vi "PicoScope4000aProbeInteraction.vi"(7 "Device Info":T2={"Driver Version"="2.1.44.2194", "USB Version"="3.0", "Hardware"="1", "Variant"="4444", "Batch and Serial"="FU827/0013", "Cal Date"="17Apr18", "Kernel Version"="1.0", "Digital HW Version"="1", "Analogue HW Version"="1", "Firmware 1"="1.7.5.0", "Firmware 2"="1.1.6.0", "Num. channels"=4}, 8 "error in":errorcluster, 11 "handle in":i16=16384) -> (0 "error out":errorcluster, 3 "handle out":i16=16384, 4 "Output Probe Array":T1(array[cluster])=[{"probeNumber"=0, FALSE, "channel"=-1, "enabled"=0, "probeName"=0, "requiresPower"=0, "isPowered"=0, "probeOff"=0, "rangeFirst"=0, "rangeLast"=0, "rangeCurrent"=0, "couplingFirst"=0, "couplingLast"=0, "couplingCurrent"=0, "filterFlags"=0, "filterCurrent"=0, "defaultFilter"=0}, {"probeNumber"=0, FALSE, "channel"=-1, "enabled"=0, "probeName"=0, "requiresPower"=0, "isPowered"=0, "probeOff"=0, "rangeFirst"=0, "rangeLast"=0, "rangeCurrent"=0, "couplingFirst"=0, "couplingLast"=0, "couplingCurrent"=0, "filterFlags"=0, "filterCurrent"=0, "defaultFilter"=0}, {"probeNumber"=0, FALSE, "channel"=-1, "enabled"=0, "probeName"=0, "requiresPower"=0, "isPowered"=0, "probeOff"=0, "rangeFirst"=0, "rangeLast"=0, "rangeCurrent"=0, "couplingFirst"=0, "couplingLast"=0, "couplingCurrent"=0, "filterFlags"=0, "filterCurrent"=0, "defaultFilter"=0}, {"probeNumber"=0, FALSE, "channel"=-1, "enabled"=0, "probeName"=0, "requiresPower"=0, "isPowered"=0, "probeOff"=0, "rangeFirst"=0, "rangeLast"=0, "rangeCurrent"=0, "couplingFirst"=0, "couplingLast"=0, "couplingCurrent"=0, "filterFlags"=0, "filterCurrent"=0, "defaultFilter"=0}], 6 "ProbeStateChanged":bool)   [LabVIEW 2010]
uses:
  ps4000aWrap.dll
panel:
  out "Probe Array Updates":T1(array[cluster])
  in  "Probe Input Array":T1(array[cluster])=[{"probeNumber"=0, FALSE, "channel"=-1, "enabled"=0, "probeName"=0, "requiresPower"=0, "isPowered"=0, "probeOff"=0, "rangeFirst"=0, "rangeLast"=0, "rangeCurrent"=0, "couplingFirst"=0, "couplingLast"=0, "couplingCurrent"=0, "filterFlags"=0, "filterCurrent"=0, "defaultFilter"=0}, {"probeNumber"=0, FALSE, "channel"=-1, "enabled"=0, "probeName"=0, "requiresPower"=0, "isPowered"=0, "probeOff"=0, "rangeFirst"=0, "rangeLast"=0, "rangeCurrent"=0, "couplingFirst"=0, "couplingLast"=0, "couplingCurrent"=0, "filterFlags"=0, "filterCurrent"=0, "defaultFilter"=0}, {"probeNumber"=0, FALSE, "channel"=-1, "enabled"=0, "probeName"=0, "requiresPower"=0, "isPowered"=0, "probeOff"=0, "rangeFirst"=0, "rangeLast"=0, "rangeCurrent"=0, "couplingFirst"=0, "couplingLast"=0, "couplingCurrent"=0, "filterFlags"=0, "filterCurrent"=0, "defaultFilter"=0}, {"probeNumber"=0, FALSE, "channel"=-1, "enabled"=0, "probeName"=0, "requiresPower"=0, "isPowered"=0, "probeOff"=0, "rangeFirst"=0, "rangeLast"=0, "rangeCurrent"=0, "couplingFirst"=0, "couplingLast"=0, "couplingCurrent"=0, "filterFlags"=0, "filterCurrent"=0, "defaultFilter"=0}]
  out "numberOfProbes":i32=1
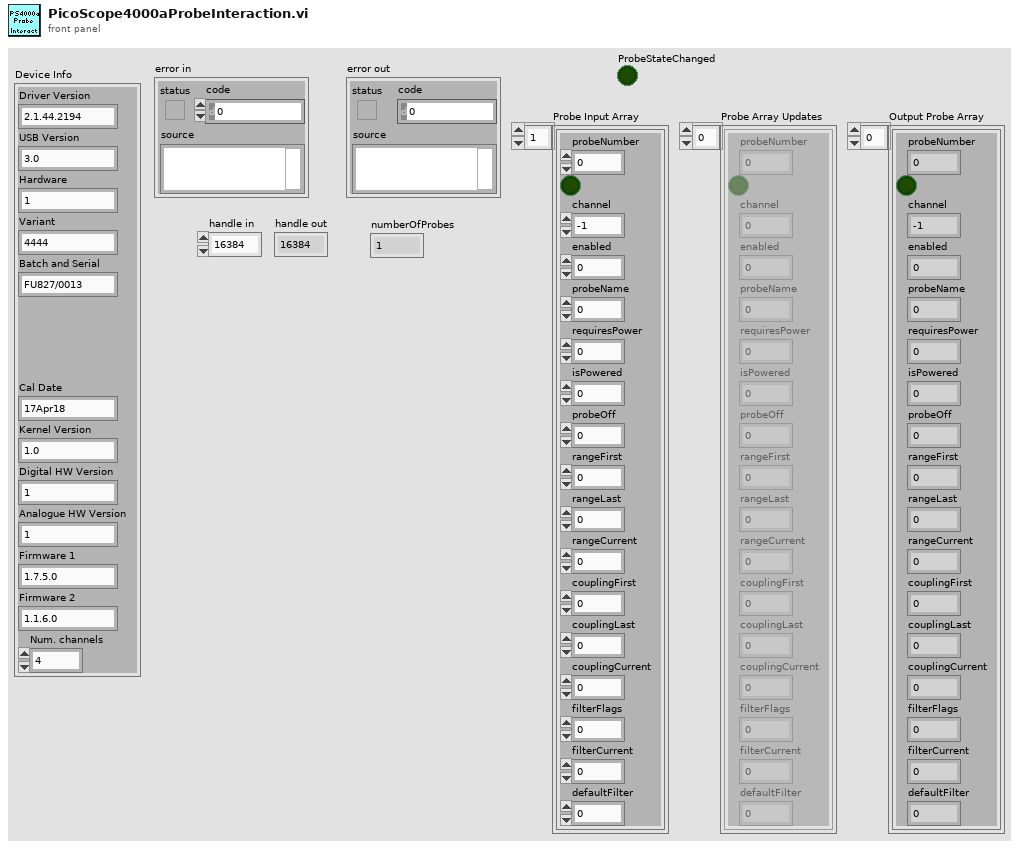
[diagram p1: front panel]
types:
  T1 = cluster{"probeNumber":i32, bool, "channel":i32, "enabled":i16, "probeName":i32, "requiresPower":i8, "isPowered":i8, "probeOff":i32, "rangeFirst":i32, "rangeLast":i32, "rangeCurrent":i32, "couplingFirst":i32, "couplingLast":i32, "couplingCurrent":i32, "filterFlags":i32, "filterCurrent":i32, "defaultFilter":i32}[]
  T2 = cluster{"Driver Version":string, "USB Version":string, "Hardware":string, "Variant":string, "Batch and Serial":string, "Cal Date":string, "Kernel Version":string, "Digital HW Version":string, "Analogue HW Version":string, "Firmware 1":string, "Firmware 2":string, "Num. channels":i16}
  T3 = cluster{"status":bool, "code":u32, "source":string}
  T4 = cluster{"probeNumber":i32, bool, "channel":i32, "enabled":i16, "probeName":i32, "requiresPower":i8, "isPowered":i8, "probeOff":i32, "rangeFirst":i32, "rangeLast":i32, "rangeCurrent":i32, "couplingFirst":i32, "couplingLast":i32, "couplingCurrent":i32, "filterFlags":i32, "filterCurrent":i32, "defaultFilter":i32}
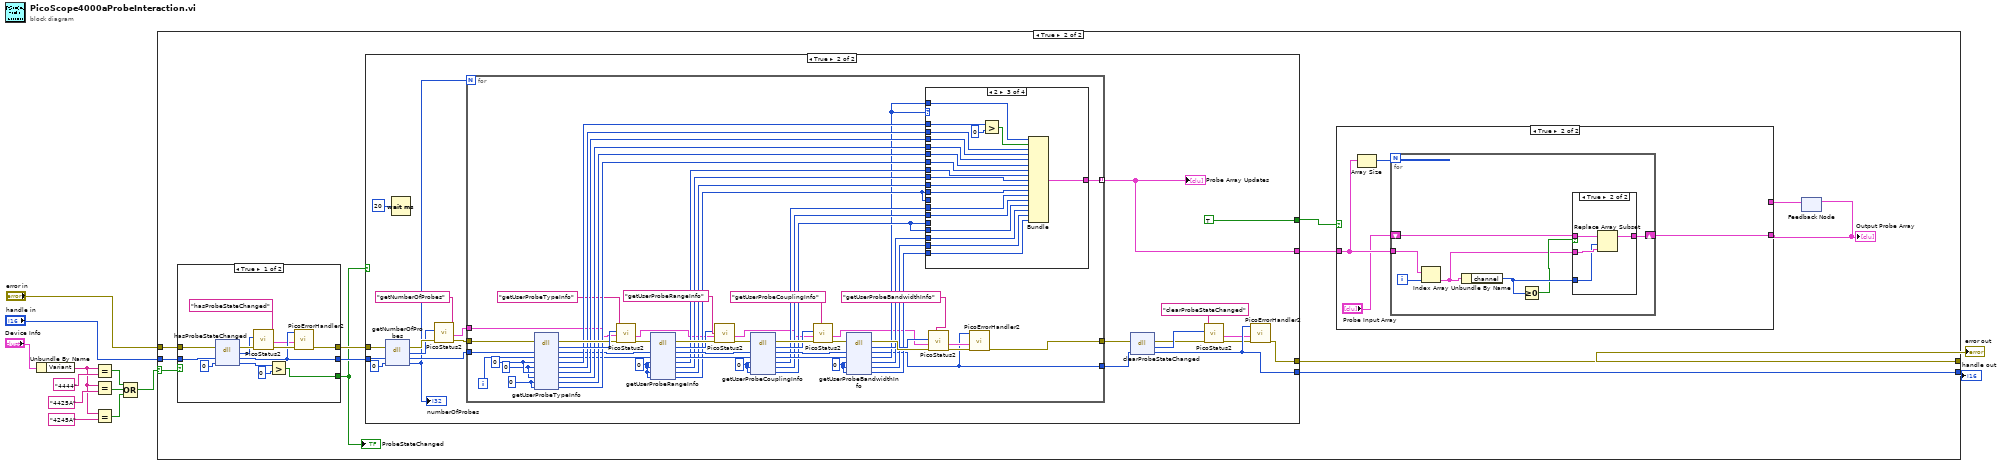
[diagram p0: block diagram]
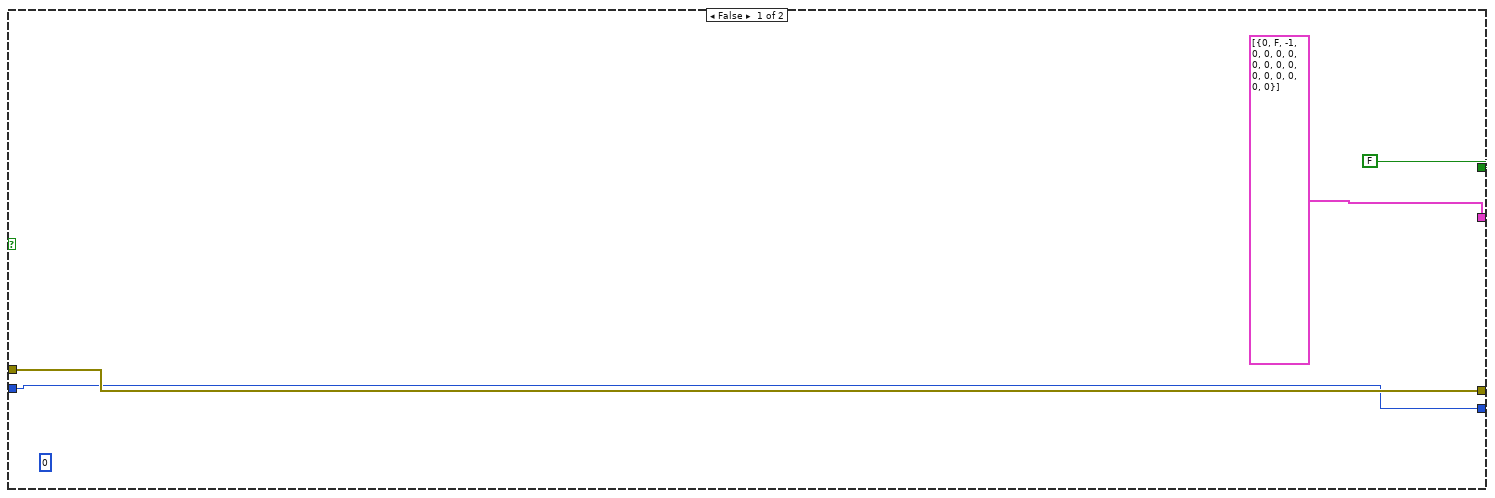
[diagram p5: hidden frame]
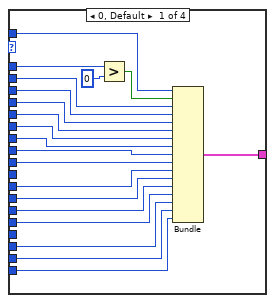
[diagram p6: hidden frame]
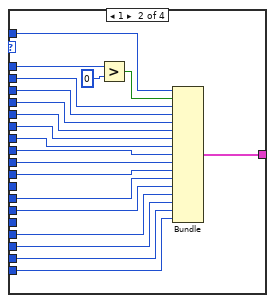
[diagram p7: hidden frame]
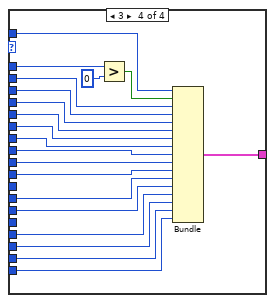
[diagram p8: hidden frame]
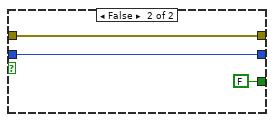
[diagram p9: hidden frame]
diagram:
  n1 = Unbundle By Name("Device Info") -> ("Variant"=w6:string)
  n2 = Equal?(x=w6, y="4444") -> (x = y?=w2:bool)
  n3 = Equal?(x=w6, y="4425A") -> (x = y?=w4:bool)
  n4 = Equal?(x=w6, y="4245A") -> (x = y?=w3:bool)
  n5 = Compound Arithmetic op=OR(w2, w4, w3) -> (w1:bool)
  n6 = case shown="True" w1 {
    selector: w1 -> [_ w20]
    tunnel: "handle in" -> [w15 w21]
    tunnel: "error in" -> [w14 w22]
    tunnel: [w14 w25] -> w13
    tunnel: [w15 w24] -> w12
    frame False {
    }
    frame True {
      n7 = case shown="True" w20 {
        tunnel: w22 -> [w219 w221]
        tunnel: w21 -> [w218 w222]
        tunnel: [w210 w221] -> w27
        tunnel: [w208 w222] -> w26
        tunnel: [w211 FALSE] -> w23
        frame True {
          n8 = dll-call lib="ps4000aWrap.dll" fn="hasProbeStateChanged"(error in=w219, "handle"=w218, "probeStateChanged"=i16 0) -> (error out=w214:errorcluster, "PICO_STATUS"=w213:u32, "handle"=w208:i16, "probeStateChanged"=w216:i16)  [unwired: 2 in, 1 out]
          n9 = call "PicoStatus2.vi"("PICO source"="hasProbeStateChanged" ("source"), "Error in"=w214, "PICO STATUS"=w213) -> ("error out"=w209:errorcluster, "PICO_STATUS out"=w207:T3)  [unwired: 5 in]
          n10 = Greater?(x=w216, y=i16 0) -> (0:w211:bool)
          n11 = call "PicoErrorHandler2.vi"("error in (no error)"=w209, "PICO_STATUS in"=w207, "handle In"=w208) -> ("error out"=w210:errorcluster)  [unwired: 8 in]
        }
        frame False {
        }
      }
      "ProbeStateChanged" <- w23
      n12 = case shown="True" w23 {
        tunnel: w27 -> [w48 w67]
        tunnel: w26 -> [w47 w66]
        tunnel: [w48 w60] -> w25
        tunnel: [w47 w57] -> w24
        tunnel: [T1 [{"probeNumber"=0, FALSE, "channel"=-1, "enabled"=0, "probeName"=0, "requiresPower"=0, "isPowered"=0, "probeOff"=0, "rangeFirst"=0, "rangeLast"=0, "rangeCurrent"=0, "couplingFirst"=0, "couplingLast"=0, "couplingCurrent"=0, "filterFlags"=0, "filterCurrent"=0, "defaultFilter"=0}] w51] -> w19
        tunnel: [FALSE TRUE] -> w18
        frame False {
          (unwired) 0 ("numberOfProbes")
        }
        frame True {
          n13 = dll-call lib="ps4000aWrap.dll" fn="getNumberOfProbes"(error in=w67, "handle"=w66, "numberOfProbes"=0) -> (error out=w70:errorcluster, "PICO_STATUS"=w69:u32, "handle"=w63:i16, "numberOfProbes"=w61:i32)  [unwired: 2 in, 1 out]
          "numberOfProbes" <- w61
          n14 = Wait (ms)(milliseconds to wait=u32 20) -> ()  [unwired: 1 out]
          n15 = call "PicoStatus2.vi"("PICO source"="getNumberOfProbes" ("source"), "Error in"=w70, "PICO STATUS"=w69) -> ("error out"=w64:errorcluster, "PICO_STATUS out"=w49:T3)  [unwired: 5 in]
          n16 = for {
            N: w61 -> [_]
            tunnel: w64 -> [w115]
            tunnel: w63 -> [w114]
            tunnel: [w76] -> w58
            tunnel: [w75] -> w59
            tunnel: [w81] -> w51 mode=indexing
            tunnel: w49 -> [w74]
            i -> [w123]
            w79 = 0 ("channel")
            w80 = i16 0 ("connected")
            w93 = 0 ("defaultFilter")
            w100 = 0 ("couplingCurrent")
            w111 = 0 ("rangeCurrent")
            w124 = i8 0 ("isPowered")
            n17 = dll-call lib="ps4000aWrap.dll" fn="getUserProbeTypeInfo"(error in=w115, "handle"=w114, "probeNumber"=w123, "connected"=w80, "channel"=w79, "enabled"=w80, "probeName"=w79, "requiresPower"=w124, "isPowered"=w124) -> (error out=w125:errorcluster, "PICO_STATUS"=w126:u32, "handle"=w113:i16, "probeNumber"=w112:i32, "connected"=w122:i16, "channel"=w117:i32, "enabled"=w121:i16, "probeName"=w118:i32, "requiresPower"=w120:i8, "isPowered"=w119:i8)  [unwired: 2 in, 1 out]
            n18 = call "PicoStatus2.vi"("PICO source"="getUserProbeTypeInfo" ("source"), "Error in"=w125, "PICO_STATUS in"=w74, "PICO STATUS"=w126) -> ("error out"=w110:errorcluster, "PICO_STATUS out"=w73:T3)  [unwired: 4 in]
            n19 = dll-call lib="ps4000aWrap.dll" fn="getUserProbeRangeInfo"(error in=w110, "handle"=w113, "probeNumber"=w112, "probeOff"=w111, "rangeFirst"=w111, "rangeLast"=w111, "rangeCurrent"=w111) -> (error out=w109:errorcluster, "PICO_STATUS"=w107:u32, "handle"=w102:i16, "probeNumber"=w101:i32, "probeOff"=w92:i32, "rangeFirst"=w91:i32, "rangeLast"=w90:i32, "rangeCurrent"=w84:i32)  [unwired: 2 in, 1 out]
            n20 = call "PicoStatus2.vi"("PICO source"="getUserProbeRangeInfo" ("source"), "Error in"=w109, "PICO_STATUS in"=w73, "PICO STATUS"=w107) -> ("error out"=w106:errorcluster, "PICO_STATUS out"=w72:T3)  [unwired: 4 in]
            n21 = dll-call lib="ps4000aWrap.dll" fn="getUserProbeCouplingInfo"(error in=w106, "handle"=w102, "probeNumber"=w101, "couplingFirst"=w100, "couplingLast"=w100, "couplingCurrent"=w100) -> (error out=w105:errorcluster, "PICO_STATUS"=w103:u32, "handle"=w95:i16, "probeNumber"=w94:i32, "couplingFirst"=w89:i32, "couplingLast"=w88:i32, "couplingCurrent"=w83:i32)  [unwired: 2 in, 1 out]
            n22 = call "PicoStatus2.vi"("PICO source"="getUserProbeCouplingInfo" ("source"), "Error in"=w105, "PICO_STATUS in"=w72, "PICO STATUS"=w103) -> ("error out"=w96:errorcluster, "PICO_STATUS out"=w71:T3)  [unwired: 4 in]
            n23 = dll-call lib="ps4000aWrap.dll" fn="getUserProbeBandwidthInfo"(error in=w96, "handle"=w95, "probeNumber"=w94, "filterFlags"=w93, "filterCurrent"=w93, "defaultFilter"=w93) -> (error out=w98:errorcluster, "PICO_STATUS"=w97:u32, "handle"=w76:i16, "probeNumber"=w82:i32, "filterFlags"=w87:i32, "filterCurrent"=w86:i32, "defaultFilter"=w85:i32)  [unwired: 2 in, 1 out]
            n24 = case shown="2" w82 {
              tunnel: w122 -> [w140 w161 w181 w201]
              tunnel: w121 -> [w146 w166 w186 w206]
              tunnel: w118 -> [w145 w165 w185 w205]
              tunnel: w120 -> [w144 w164 w184 w204]
              tunnel: w119 -> [w143 w163 w183 w203]
              tunnel: w117 -> [w142 w162 w182 w202]
              tunnel: w92 -> [w138 w157 w177 w197]
              tunnel: w91 -> [w137 w156 w176 w196]
              tunnel: w90 -> [w136 w155 w175 w195]
              tunnel: w84 -> [w135 _ _ _]
              tunnel: w89 -> [w134 w153 w173 w193]
              tunnel: w88 -> [w133 w152 w172 w192]
              tunnel: w83 -> [w132 _ _ _]
              tunnel: w87 -> [w131 w150 w170 w190]
              tunnel: w86 -> [w130 w149 w169 w189]
              tunnel: w85 -> [w129 w148 w168 w188]
              tunnel: w82 -> [w128 w158 w178 w198]
              tunnel: w84 -> [_ w154 w174 w194]
              tunnel: w83 -> [_ w151 w171 w191]
              tunnel: [w127 w147 w167 w187] -> w81
              frame 0, Default {
                n25 = Greater?(x=w140, y=i16 0) -> (0:w139:bool)
                n26 = Bundle("probeNumber"=w128, w139, "channel"=w142, "enabled"=w146, "probeName"=w145, "requiresPower"=w144, "isPowered"=w143, "probeOff"=w138, "rangeFirst"=w137, "rangeLast"=w136, "rangeCurrent"=w135, "couplingFirst"=w134, "couplingLast"=w133, "couplingCurrent"=w132, "filterFlags"=w131, "filterCurrent"=w130, "defaultFilter"=w129) -> (w127:T4)  [unwired: 1 in]
              }
              frame 1 {
                n27 = Greater?(x=w161, y=i16 0) -> (0:w159:bool)
                n28 = Bundle("probeNumber"=w158, w159, "channel"=w162, "enabled"=w166, "probeName"=w165, "requiresPower"=w164, "isPowered"=w163, "probeOff"=w157, "rangeFirst"=w156, "rangeLast"=w155, "rangeCurrent"=w154, "couplingFirst"=w153, "couplingLast"=w152, "couplingCurrent"=w151, "filterFlags"=w150, "filterCurrent"=w149, "defaultFilter"=w148) -> (w147:T4)  [unwired: 1 in]
              }
              frame 2 {
                n29 = Greater?(x=w181, y=i16 0) -> (0:w179:bool)
                n30 = Bundle("probeNumber"=w178, w179, "channel"=w182, "enabled"=w186, "probeName"=w185, "requiresPower"=w184, "isPowered"=w183, "probeOff"=w177, "rangeFirst"=w176, "rangeLast"=w175, "rangeCurrent"=w174, "couplingFirst"=w173, "couplingLast"=w172, "couplingCurrent"=w171, "filterFlags"=w170, "filterCurrent"=w169, "defaultFilter"=w168) -> (w167:T4)  [unwired: 1 in]
              }
              frame 3 {
                n31 = Greater?(x=w201, y=i16 0) -> (0:w199:bool)
                n32 = Bundle("probeNumber"=w198, w199, "channel"=w202, "enabled"=w206, "probeName"=w205, "requiresPower"=w204, "isPowered"=w203, "probeOff"=w197, "rangeFirst"=w196, "rangeLast"=w195, "rangeCurrent"=w194, "couplingFirst"=w193, "couplingLast"=w192, "couplingCurrent"=w191, "filterFlags"=w190, "filterCurrent"=w189, "defaultFilter"=w188) -> (w187:T4)  [unwired: 1 in]
              }
            }
            n33 = call "PicoStatus2.vi"("PICO source"="getUserProbeBandwidthInfo" ("source"), "Error in"=w98, "PICO_STATUS in"=w71, "PICO STATUS"=w97) -> ("error out"=w77:errorcluster, "PICO_STATUS out"=w78:T3)  [unwired: 4 in]
            n34 = call "PicoErrorHandler2.vi"("error in (no error)"=w77, "PICO_STATUS in"=w78, "handle In"=w76) -> ("error out"=w75:errorcluster)  [unwired: 8 in]
          }
          "Probe Array Updates" <- w51
          n35 = dll-call lib="ps4000aWrap.dll" fn="clearProbeStateChanged"(error in=w59, "handle"=w58) -> (error out=w53:errorcluster, "PICO_STATUS"=w54:u32, "handle"=w57:i16)  [unwired: 2 in, 1 out]
          n36 = call "PicoStatus2.vi"("PICO source"="clearProbeStateChanged" ("source"), "Error in"=w53, "PICO STATUS"=w54) -> ("error out"=w55:errorcluster, "PICO_STATUS out"=w50:T3)  [unwired: 5 in]
          n37 = call "PicoErrorHandler2.vi"("error in (no error)"=w55, "PICO_STATUS in"=w50, "handle In"=w57) -> ("error out"=w60:errorcluster)  [unwired: 8 in]
        }
      }
      n38 = feedback #1() -> (w17:T1)  [unwired: 1 in]
      n39 = case shown="True" w18 {
        tunnel: w19 -> [_ w31]
        tunnel: [w28 w29] -> w16
        tunnel: w17 -> [w28 _]
        frame False {
        }
        frame True {
          n40 = Array Size(array=w31) -> (size(s)=w32:i32)
          n41 = for {
            N: w32 -> [_]
            tunnel: w31 -> [w38]
            shift-right: [w36] -> w29
            shift-left: "Probe Input Array" -> [w33]
            i -> [w39]
            n42 = Index Array(array=w38, index=w39) -> (element=w34:T4)
            n43 = Unbundle By Name(w34) -> ("channel"=w37:i32)
            n44 = Greater Or Equal To 0?(x=w37) -> (x >= 0?=w35:bool)
            n45 = case shown="True" w35 {
              tunnel: w34 -> [_ w44]
              tunnel: w37 -> [_ w43]
              tunnel: [w40 w42] -> w36
              tunnel: w33 -> [w40 w41]
              frame False {
              }
              frame True {
                n46 = Replace Array Subset(array=w41, new element=w44, index=w43) -> (w42:T1)
              }
            }
          }
        }
      }
      "Output Probe Array" <- w16
      n47 = feedback-in #1(w16) -> ()
    }
  }
  "error out" <- w13
  "handle out" <- w12
